vi "MULTTCP2_Is_Callback.vi"(8 "error in (no error)":errorcluster, 10 "Connections":string) -> (0 "error out":errorcluster, 2 "callback?":bool)   [LabVIEW 2016]
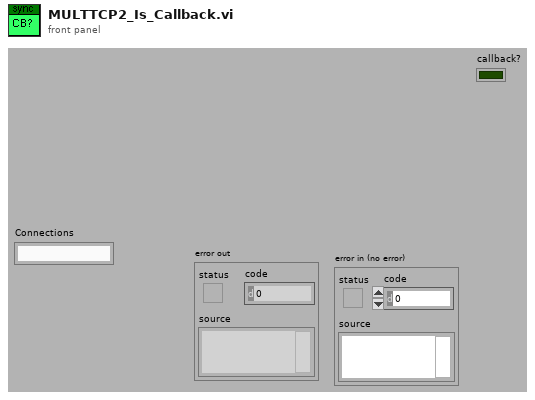
[diagram p1: front panel]
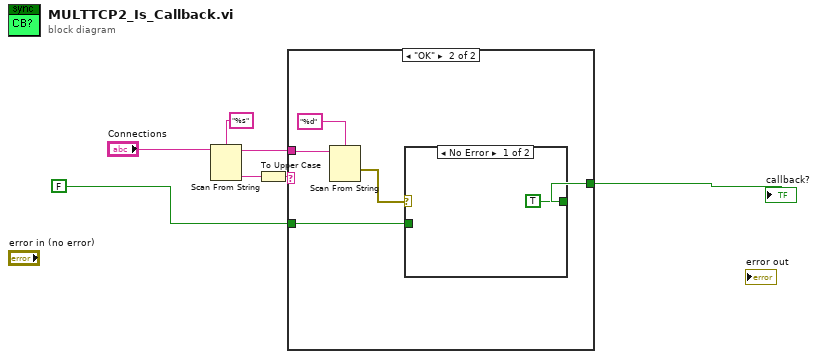
[diagram p0: block diagram]
diagram:
  n1 = Scan From String(format string="%s", input string="Connections") -> (remaining string=w3:string, output 1=w1:string)  [unwired: 2 in, 3 out]
  n2 = To Upper Case(1:w1) -> (0:w4:string)
  n3 = case shown="\"OK\"" w4 {
    tunnel: w3 -> [_ w11]
    tunnel: [w8 w13] -> w6
    tunnel: FALSE -> [w8 w12]
    frame Default {
    }
    frame "OK" {
      n4 = Scan From String(format string="%d", input string=w11) -> (error out=w9:errorcluster)  [unwired: 2 in, 4 out]
      n5 = case shown="No Error" w9 {
        tunnel: [TRUE w15] -> w13
        tunnel: w12 -> [_ w15]
        frame No Error {
        }
        frame Error {
        }
      }
    }
  }
  "callback?" <- w6
